vi "Write Resource Data ref.vi"(8 "error in (no error)":errorcluster, 10 "Resource Data ref":refnum<data-value>, 11 "Project Data in":refnum<class "Project Data.lvclass">) -> (0 "error out":errorcluster, 3 "Project Data out":refnum<class "Project Data.lvclass">)   [LabVIEW 2013, in "SET Project Data.lvlib" / "Project Data.lvclass"]
uses:
  Project Data.lvclass
  Resource Data Class/Resource Data.lvclass
  Project Data.lvclass/Project Data.ctl
  Menu Class/Menu Data.lvclass/Menu Data.ctl
  Menu Class/Menu Data.lvclass
  VI Class/VI Data.lvclass
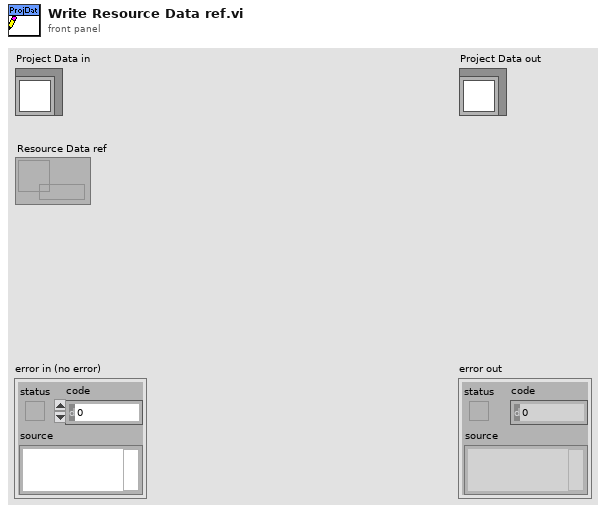
[diagram p1: front panel]
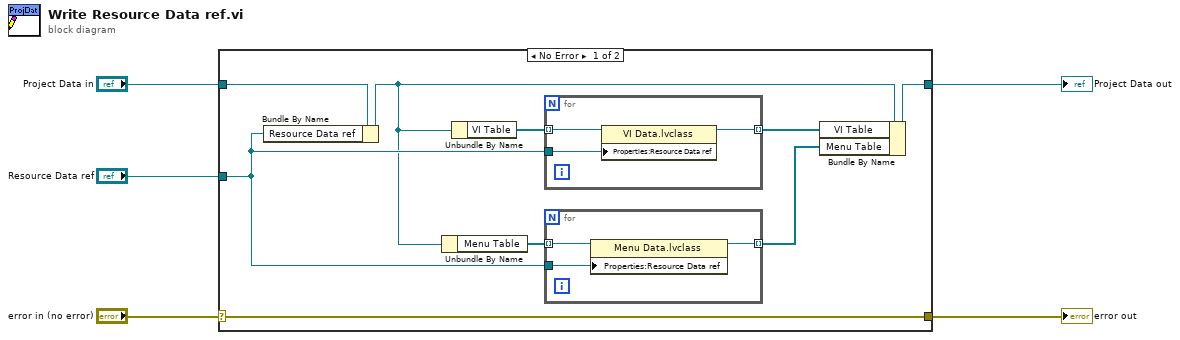
[diagram p0: block diagram]
diagram:
  n1 = case shown="No Error" "error in (no error)" {
    selector: "error in (no error)" -> [w14 w21]
    tunnel: [w14 w21] -> w4
    tunnel: [w8 w22] -> w2
    tunnel: "Project Data in" -> [w13 w22]
    tunnel: "Resource Data ref" -> [w10 _]
    frame No Error {
      n2 = Bundle By Name(cluster=w13, "Resource Data ref"=w10) -> (w9:refnum<class "Project Data.lvclass">)
      n3 = Unbundle By Name(w9) -> ("Menu Table"=w11:refnum<class "Menu Data.lvclass">[])
      n4 = Unbundle By Name(w9) -> ("VI Table"=w12:refnum<class "VI Data.lvclass">[])
      n5 = for {
        tunnel: w12 -> [w20] mode=indexing
        tunnel: w10 -> [w19]
        tunnel: [w18] -> w7 mode=indexing
        n6 = property class="VI Data.lvclass"(reference=w20, "Properties:Resource Data ref"=w19) -> (reference out=w18:refnum<class "VI Data.lvclass">)  [unwired: 1 in, 1 out]
      }
      n7 = for {
        tunnel: w11 -> [w17] mode=indexing
        tunnel: w10 -> [w16]
        tunnel: [w15] -> w6 mode=indexing
        n8 = property class="Menu Data.lvclass"(reference=w17, "Properties:Resource Data ref"=w16) -> (reference out=w15:refnum<class "Menu Data.lvclass">)  [unwired: 1 in, 1 out]
      }
      n9 = Bundle By Name(cluster=w9, "VI Table"=w7, "Menu Table"=w6) -> (w8:refnum<class "Project Data.lvclass">)
    }
    frame Error {
    }
  }
  "error out" <- w4
  "Project Data out" <- w2
